vi "Read Serial - host.vi"(8 "Term Char":string, 9 "Timeout (ms)":i32, 11 "Refnum in":T1) -> (2 "String out":string, 3 "Reference Out":T1, 4 "Elements Remaining":u32)   [LabVIEW 2012]
uses:
  FPGA_ref.ctl
  <vilib>/Utility/error.llb/Error Cluster From Error Code.vi
  <vilib>/rvi/errors/niLvFpgaAdjustHostInterfaceError.vi
  <vilib>/rvi/interface/nirviMethod/nirviMethod.xnode
  <vilib>/FPGAPlugInAG/Dynamic/niLvFpga_ReadFifo_Dynamic.vi
  <vilib>/rvi/errors/niLvFpgaMergeErrorWithErrorCode.vi
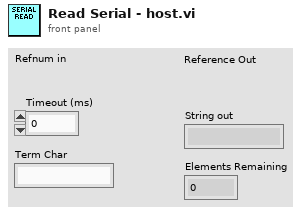
[diagram p1: front panel]
types:
  T1 = typedef "FPGA_ref.ctl" = refnum<k20>
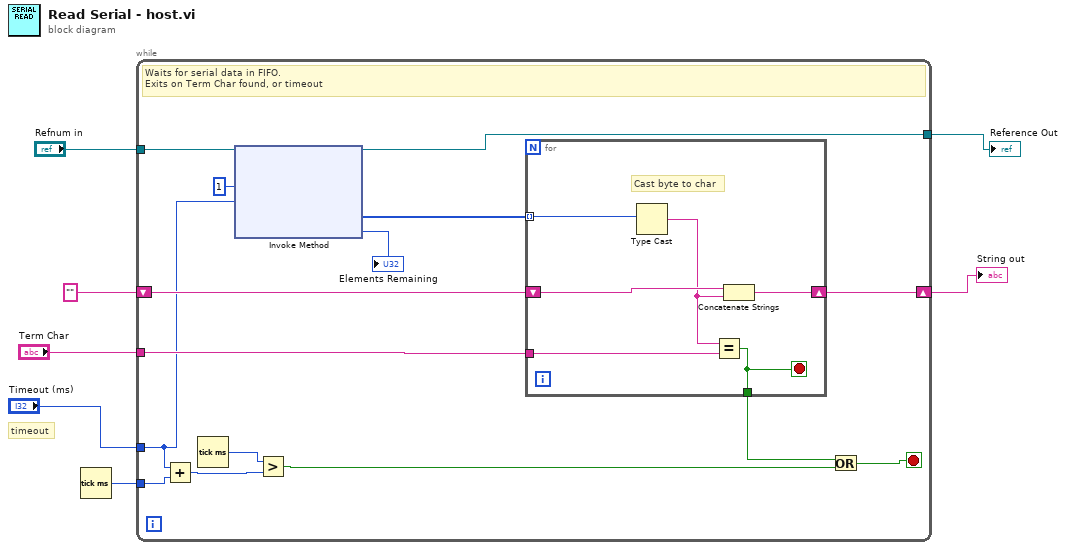
[diagram p0: block diagram]
diagram:
  # "timeout"
  n1 = Tick Count (ms)() -> (millisecond timer value=w3:u32)
  n2 = while {
    tunnel: "Refnum in" -> [w11]
    tunnel: "Term Char" -> [w16]
    tunnel: "Timeout (ms)" -> [w10]
    tunnel: w3 -> [w19]
    shift-right: [w22] -> w7
    shift-left: "" -> [w14]
    tunnel: [w8] -> w1
    stop <- w21 stop-if-true
    # "Waits for serial data in FIFO.\nExits on Term Char found, or timeout"
    n3 = Add(x=w10, y=w19) -> (x+y=w18:u32)
    n4 = Tick Count (ms)() -> (millisecond timer value=w20:u32)
    n5 = xnode "Invoke Method"("FPGA VI Reference In"=w11, "Number of Elements"=u32 1, "Timeout (ms)"=w10) -> ("FPGA VI Reference Out"=w8:T1, "Data"=w12:u8[], "Elements Remaining"=→"Elements Remaining":u32)  [unwired: 1 in, 1 out]
    n6 = Greater?(x=w20, y=w18) -> (0:w17:bool)
    n7 = for {
      tunnel: w12 -> [w28] mode=indexing
      tunnel: w16 -> [w27]
      tunnel: [w23] -> w15
      shift-right: [w24] -> w22
      shift-left: w14 -> [w26]
      stop <- w23 stop-if-true
      # "Cast byte to char"
      n8 = Type Cast(x=w28) -> (*(type *) &x=w25:string)  [unwired: 1 in]
      n9 = Equal?(x=w25, y=w27) -> (x = y?=w23:bool)
      n10 = Concatenate Strings(w26, w25) -> (w24:string)
    }
    n11 = Or(x=w15, y=w17) -> (x .or. y?=w21:bool)
  }
  "String out" <- w7
  "Reference Out" <- w1
